vi "AlliGator Remove Keywords from Action String.vi"(8 "error in (no error)":errorcluster, 11 "String":string) -> (0 "error out":errorcluster, 3 "String w/o keywords":string)   [LabVIEW 2021, in "AlliGator Notebook.lvlib"]
doc: "Removes frequent internal events from list of printed events in verbose mode."
uses:
  AlliGator Notebook.lvlib
panel:
  # "see the AlliGator License on the block diagram (Ctrl+E or Window:Show Block Diagram)"
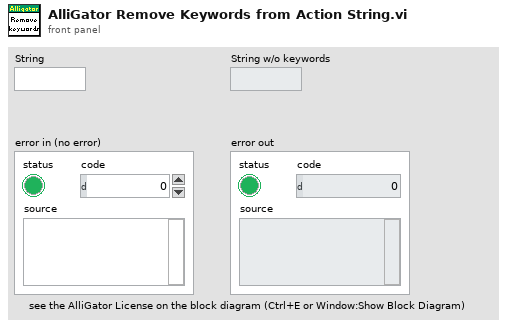
[diagram p1: front panel]
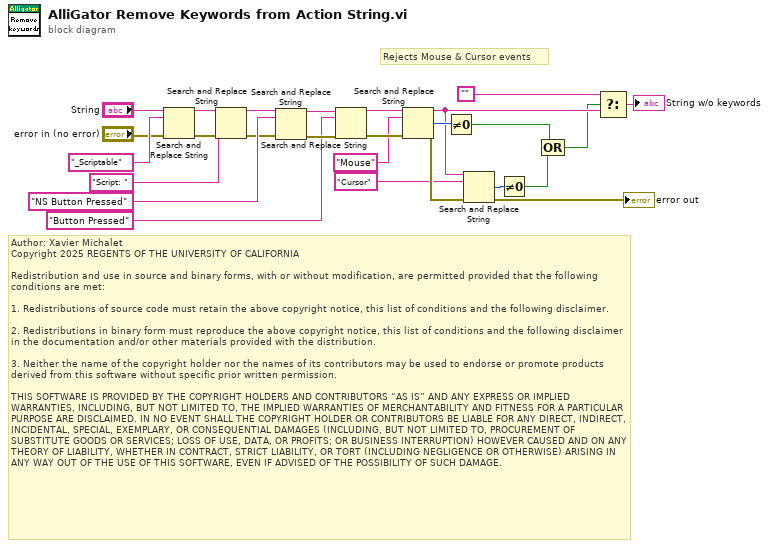
[diagram p0: block diagram]
diagram:
  # "Author: Xavier Michalet\nCopyright 2025 REGENTS OF THE UNIVERSITY OF CALIFORNIA\n\nRedistribution and use in source and binary forms, with or without modification, are permitted provided that the following conditions are met:\n\n1. Redistributions of source code must retain the above copyright notice, this list of conditions and the following disclaimer.\n\n2. Redistributions in binary form must reproduce the above copyright notice, this list of conditions and the following disclaimer in the documentation and/or other materials provided with the distribution.\n\n3. Neither the name of the copyright holder nor the names of its contributors may be used to endorse or promote products derived from this software without specific prior written permission.\n\nTHIS SOFTWARE IS PROVIDED BY THE COPYRIGHT HOLDERS AND CONTRIBUTORS “AS IS” AND ANY EXPRESS OR IMPLIED WARRANTIES, INCLUDING, BUT NOT LIMITED TO, THE IMPLIED WARRANTIES OF MERCHANTABILITY AND FITNESS FOR A PARTICULAR PURPOSE ARE DISCLAIMED. IN NO EVENT SHALL THE COPYRIGHT HOLDER OR CONTRIBUTORS BE LIABLE FOR ANY DIRECT, INDIRECT, INCIDENTAL, SPECIAL, EXEMPLARY, OR CONSEQUENTIAL DAMAGES (INCLUDING, BUT NOT LIMITED TO, PROCUREMENT OF SUBSTITUTE GOODS OR SERVICES; LOSS OF USE, DATA, OR PROFITS; OR BUSINESS INTERRUPTION) HOWEVER CAUSED AND ON ANY THEORY OF LIABILITY, WHETHER IN CONTRACT, STRICT LIABILITY, OR TORT (INCLUDING NEGLIGENCE OR OTHERWISE) ARISING IN ANY WAY OUT OF THE USE OF THIS SOFTWARE, EVEN IF ADVISED OF THE POSSIBILITY OF SUCH DAMAGE."
  # "Rejects Mouse & Cursor events"
  n1 = Search and Replace String(input string="String", search string="_Scriptable" ("substring (\"\")"), error in="error in (no error)") -> (result string=w24:string, error out=w25:errorcluster)  [unwired: 5 in, 2 out]
  n2 = Search and Replace String(input string=w24, search string="Script: " ("substring (\"\")"), error in=w25) -> (result string=w17:string, error out=w18:errorcluster)  [unwired: 5 in, 2 out]
  n3 = Search and Replace String(input string=w17, search string="NS Button Pressed" ("substring (\"\")"), error in=w18) -> (result string=w19:string, error out=w20:errorcluster)  [unwired: 5 in, 2 out]
  n4 = Search and Replace String(input string=w19, search string="Button Pressed" ("substring (\"\")"), error in=w20) -> (result string=w13:string, error out=w14:errorcluster)  [unwired: 5 in, 2 out]
  n5 = Search and Replace String(input string=w13, search string="Mouse", error in=w14) -> (result string=w6:string, number of replacements=w11:i32, error out=w7:errorcluster)  [unwired: 5 in, 1 out]
  n6 = Not Equal To 0?(x=w11) -> (x != 0?=w10:bool)
  n7 = Search and Replace String(input string=w6, search string="Cursor", error in=w7) -> (number of replacements=w4:i32, error out=→"error out":errorcluster)  [unwired: 5 in, 2 out]
  n8 = Not Equal To 0?(x=w4) -> (x != 0?=w1:bool)
  n9 = Compound Arithmetic op=OR(w10, w1) -> (w3:bool)
  n10 = Select(t="", s=w3, f=w6) -> (s? t:f=→"String w/o keywords":string)
